vi "Get Reference.vi"(8 "Error In":errorcluster, 9 "Subpanel Ref":refnum<vi>, 11 "INL DNL Test in":refnum<class "INL DNL Test.lvclass">) -> (0 "Error Out":errorcluster, 3 "INL DNL Test out":refnum<class "INL DNL Test.lvclass">)   [LabVIEW 2020, in "INL DNL Test.lvclass"]
uses:
  INL DNL Test.lvclass
  D:/INL DNL Test/Class/Test/Parent/Test.lvclass
  Parent/Typedef/LV2 Control.ctl
  Device/Parent/Device.lvclass
  Parent/Test.lvclass
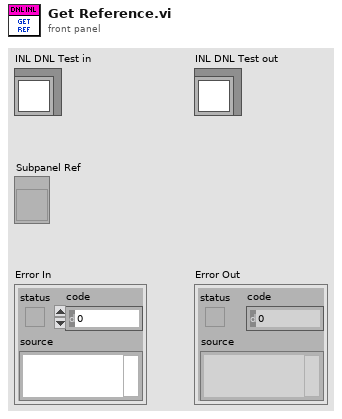
[diagram p1: front panel]
types:
  T1 = typedef "Test.lvclass/LV2 Control.ctl" = enum16{"Home", "Mode", "Config", "Status", "Read"}
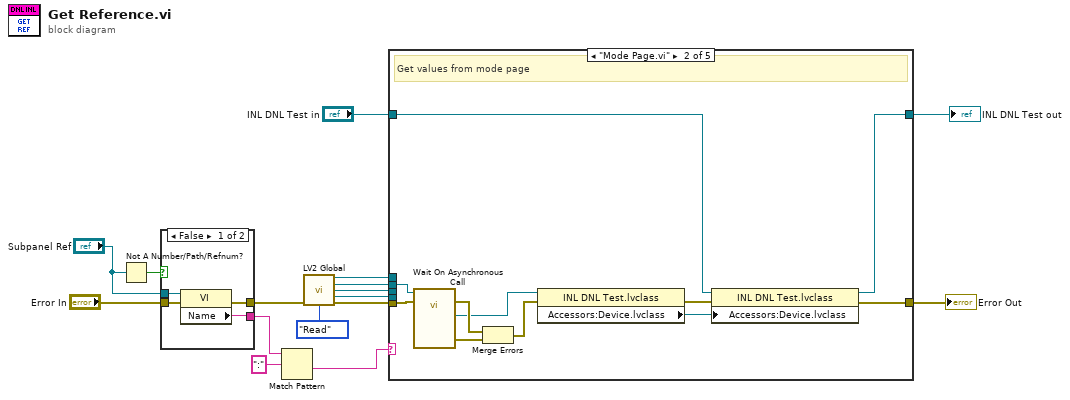
[diagram p0: block diagram]
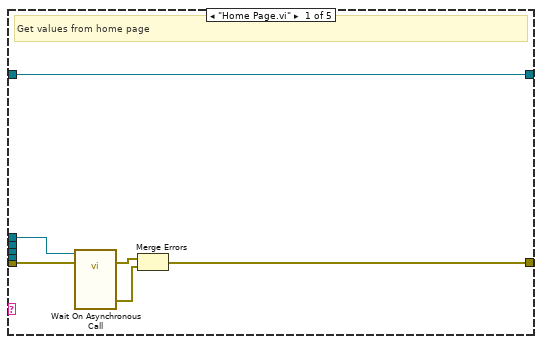
[diagram p2: hidden frame]
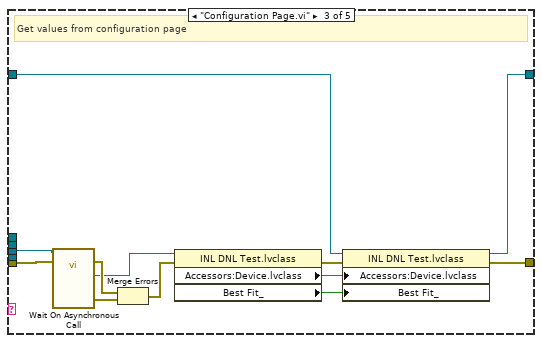
[diagram p3: hidden frame]
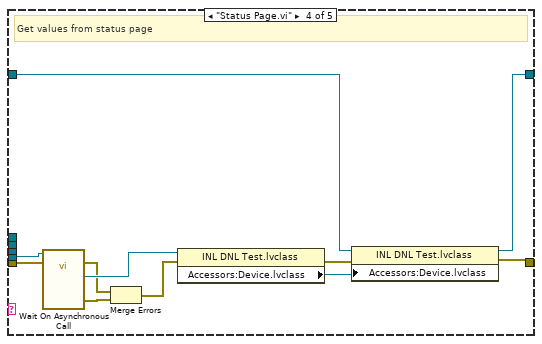
[diagram p4: hidden frame]
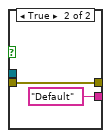
[diagram p6: hidden frame]
diagram:
  n1 = Not A Number/Path/Refnum?(number/path/refnum="Subpanel Ref") -> (NaN/Path/Refnum?=w15:bool)
  n2 = case shown="False" w15 {
    tunnel: "Error In" -> [w20 w22]
    tunnel: [w19 w22] -> w12
    tunnel: [w18 "Default" ("Name")] -> w4
    tunnel: "Subpanel Ref" -> [w17 _]
    frame False {
      n3 = property class="VI"(reference=w17, error in=w20) -> (error out=w19:errorcluster, "Name"=w18:string)  [unwired: 1 out]
    }
    frame True {
    }
  }
  n4 = Match Pattern(string=w4, regular expression=":") -> (after substring=w2:string)  [unwired: 1 in, 3 out]
  n5 = call "LV2 Global.vi"("Error In"=w12, "Enum"=LV2_Control."Read") -> ("Home Ref"=w1:refnum<vi>, "Mode Ref"=w7:refnum<vi>, "Config Ref"=w8:refnum<vi>, "Status Ref"=w9:refnum<vi>, "Error Out"=w11:errorcluster)  [unwired: 9 in]
  n6 = case shown="\"Mode Page.vi\"" w2 {
    tunnel: w11 -> [w26 w39 w48 w62 w64]
    tunnel: [w23 w35 w44 w55 w64] -> w13
    tunnel: w9 -> [_ _ _ w54 _]
    tunnel: w8 -> [_ _ w42 _ _]
    tunnel: w7 -> [_ w31 _ _ _]
    tunnel: [w28 w29 w40 w52 w63] -> w5
    tunnel: "INL DNL Test in" -> [w28 w30 w41 w53 w63]
    tunnel: w1 -> [w27 _ _ _ _]
    frame "Home Page.vi" {
      # "Get values from home page"
      n7 = call-by-ref "Wait On Asynchronous Call"(reference=w27, error in=w26) -> (error out=w25:errorcluster, "Error Out"=w24:errorcluster)  [unwired: 14 in, 2 out]
      n8 = Merge Errors(w25, w24) -> (w23:errorcluster)
    }
    frame "Mode Page.vi" {
      # "Get values from mode page"
      n9 = call-by-ref "Wait On Asynchronous Call"(reference=w31, error in=w39) -> (error out=w38:errorcluster, "Error out"=w37:errorcluster, "reference out"=w33:refnum<class "INL DNL Test.lvclass">)  [unwired: 10 in, 1 out]
      n10 = Merge Errors(w38, w37) -> (w36:errorcluster)
      n11 = property class="INL DNL Test.lvclass"(reference=w33, error in=w36) -> (error out=w34:errorcluster, "Accessors:Device.lvclass"=w32:refnum<class "Device.lvclass">)  [unwired: 1 out]
      n12 = property class="INL DNL Test.lvclass"(reference=w30, error in=w34, "Accessors:Device.lvclass"=w32) -> (reference out=w29:refnum<class "INL DNL Test.lvclass">, error out=w35:errorcluster)
    }
    frame "Configuration Page.vi" {
      # "Get values from configuration page"
      n13 = call-by-ref "Wait On Asynchronous Call"(reference=w42, error in=w48) -> (error out=w47:errorcluster, "Error out"=w46:errorcluster, "INL DNL Test.lvclass 2"=w45:refnum<class "INL DNL Test.lvclass">)  [unwired: 10 in, 1 out]
      n14 = Merge Errors(w47, w46) -> (w51:errorcluster)
      n15 = property class="INL DNL Test.lvclass"(reference=w45, error in=w51) -> (error out=w50:errorcluster, "Accessors:Device.lvclass"=w49:refnum<class "Device.lvclass">, "Best Fit_"=w43:bool)  [unwired: 1 out]
      n16 = property class="INL DNL Test.lvclass"(reference=w41, error in=w50, "Accessors:Device.lvclass"=w49, "Best Fit_"=w43) -> (reference out=w40:refnum<class "INL DNL Test.lvclass">, error out=w44:errorcluster)
    }
    frame "Status Page.vi" {
      # "Get values from status page"
      n17 = call-by-ref "Wait On Asynchronous Call"(reference=w54, error in=w62) -> (error out=w59:errorcluster, "Error out"=w60:errorcluster, "INL DNL Test out"=w61:refnum<class "INL DNL Test.lvclass">)  [unwired: 10 in, 1 out]
      n18 = Merge Errors(w59, w60) -> (w58:errorcluster)
      n19 = property class="INL DNL Test.lvclass"(reference=w61, error in=w58) -> (error out=w57:errorcluster, "Accessors:Device.lvclass"=w56:refnum<class "Device.lvclass">)  [unwired: 1 out]
      n20 = property class="INL DNL Test.lvclass"(reference=w53, error in=w57, "Accessors:Device.lvclass"=w56) -> (reference out=w52:refnum<class "INL DNL Test.lvclass">, error out=w55:errorcluster)
    }
    frame Default {
      # "Default state"
    }
  }
  "Error Out" <- w13
  "INL DNL Test out" <- w5
